vi "DSF.Engine.Memory.Pointer.DataType.New.vi"(8 "error in (no error)":errorcluster, 11 "count (1)":u64=1 format="%d elements") -> (0 "error out":errorcluster, 3 "Data Type pointer":refnum<class "DSF.Engine.Memory.Pointer.DataType.lvclass">)   [LabVIEW 2016, in "DSF.Engine.lvlib" / "DSF.Engine.Memory.Pointer.DataType.lvclass"]
uses:
  DSF.Engine.Memory.Pointer.DataType.lvclass
  C:/Git/Sourcetree/DSF/Source/Submodules/Memory/Source/Classes/Internal/Memory.Pointer.Internal.lvclass
  Submodules/Memory/Source/Classes/Internal/Memory.Pointer.Internal.lvclass
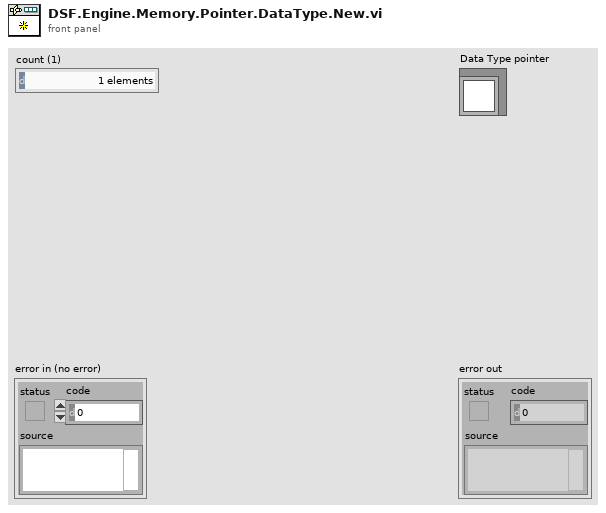
[diagram p1: front panel]
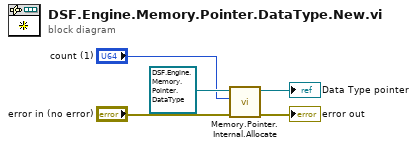
[diagram p0: block diagram]
diagram:
  n1 = call "Memory.Pointer.Internal.Allocate.vi"("error in (no error)"="error in (no error)", "size"="count (1)", "pointer in"=refnum<class "DSF.Engine.Memory.Pointer.DataType.lvclass"> refnum ("DSF.Memory.Pointer.Data Type in")) -> ("error out"=→"error out":errorcluster, "pointer out"=→"Data Type pointer":refnum<class "DSF.Engine.Memory.Pointer.DataType.lvclass">)  [unwired: 7 in]
